vi "HMI.vi"(8 "error in (no error)":errorcluster caption="entrée d'erreur (pas d'erreur)", 11 "Class Popup WaitDIO en entrée":refnum<class "Class Popup WaitVoltage.lvclass">) -> (0 "error out":errorcluster caption="sortie d'erreur", 1 "Input":string, 2 "Operator_Selection":bool, 3 "Class Popup WaitDIO en sortie":refnum<class "Class Popup WaitVoltage.lvclass">)   [LabVIEW 2020, in "Library Instrument & Equipement.lvlib" / "Library Popup.lvlib" / "Class Popup WaitVoltage.lvclass"]
uses:
  Class Popup WaitVoltage.lvclass
  C:/Users/ngarcin/OneDrive - Altyor/Standard TB/Class/Popup/Class Popup (Main)/Class Popup (Main).lvclass
  C:/Users/ngarcin/OneDrive - Altyor/Standard TB/Class/Popup/Class Popup Operator_Validation/Class Popup Operator_Validation (Default)/Class Popup Operator_Validation (Virtual).lvclass
  Commun VI/TypeDef/Liste Error.ctl
  JSON API/JSON Value/Set from JSON string.vi
  Instrument/Instrument (Default)/Class Instrument (Default).lvclass
  JSON API/JSON Value/JSON Value.lvclass
  Class Popup Operator_Validation/Class Popup Operator_Validation (Default)/Class Popup Operator_Validation (Virtual).lvclass
  Class Popup WaitVoltage.lvclass/Class Popup WaitVoltage.ctl
  JSON API/Variant JSON/Variant JSON.lvlib
  JSON API/Get Polymorphic/JSON GetSet.lvlib
  Commun VI/Library Commun.lvlib
panel:
  out "Voltage":dbl format="%#.3g"
  out "Json_String":string
  in  "Bouton NOK":bool caption="Default"
  in  "Bouton OK":bool caption="Validated"
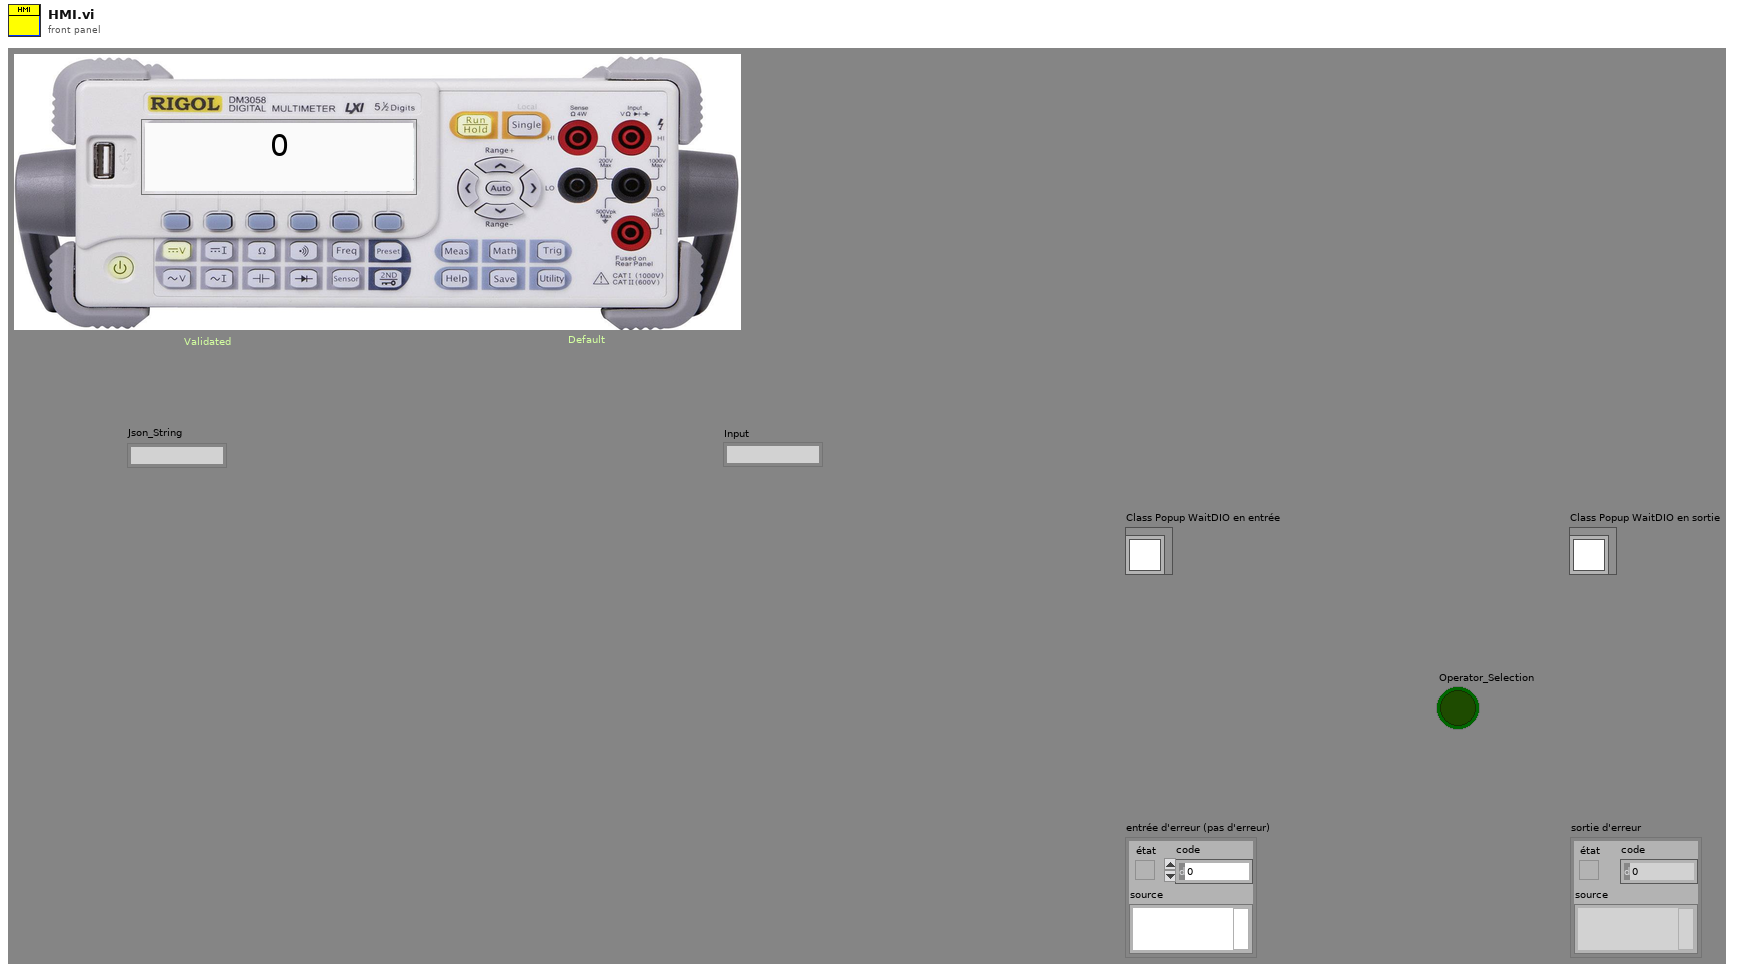
[diagram p1: front panel]
types:
  T1 = cluster{"Instrument":refnum<class "Class Instrument (Default).lvclass">, "Timeout (ms)":u64, "Value Max":dbl, "Value Min":dbl}
  T2 = typedef "Library Commun.lvlib/Liste Error.ctl" = enum16{"Firebase Driver - Get Document", "Firebase Driver - Get Document With Where", "Firebase Driver - Delete Document", "Firebase Driver - Set Document", "Firebase Driver - Update Document", "Firebase Altyor - Search Document Bench", "Firebase Altyor - Class Not in Firebase", "Spectrum_Analyser - Timeout", "Relay Board - Qty Relay", "DIO - Pb Funtion", "Power_Supply - Peripherical not find", "Mutimeter - Peripherical not find", "Instrument - Function Not Used", "Instrument - Instrument name not specified", "Instrument - Allready Initialised", "Instrument - TimeOut", "Instrument - the instrument must be Initialise before", "Instrument - Frame Not received", "Instrument - Frame Nok", "Test - Initialise the File_for_Save", "Test - Timeout", "Test - Cmd Error", "FGV - Variable ", "BDD FireBase - Define Class", "SN - Class Not Define"}
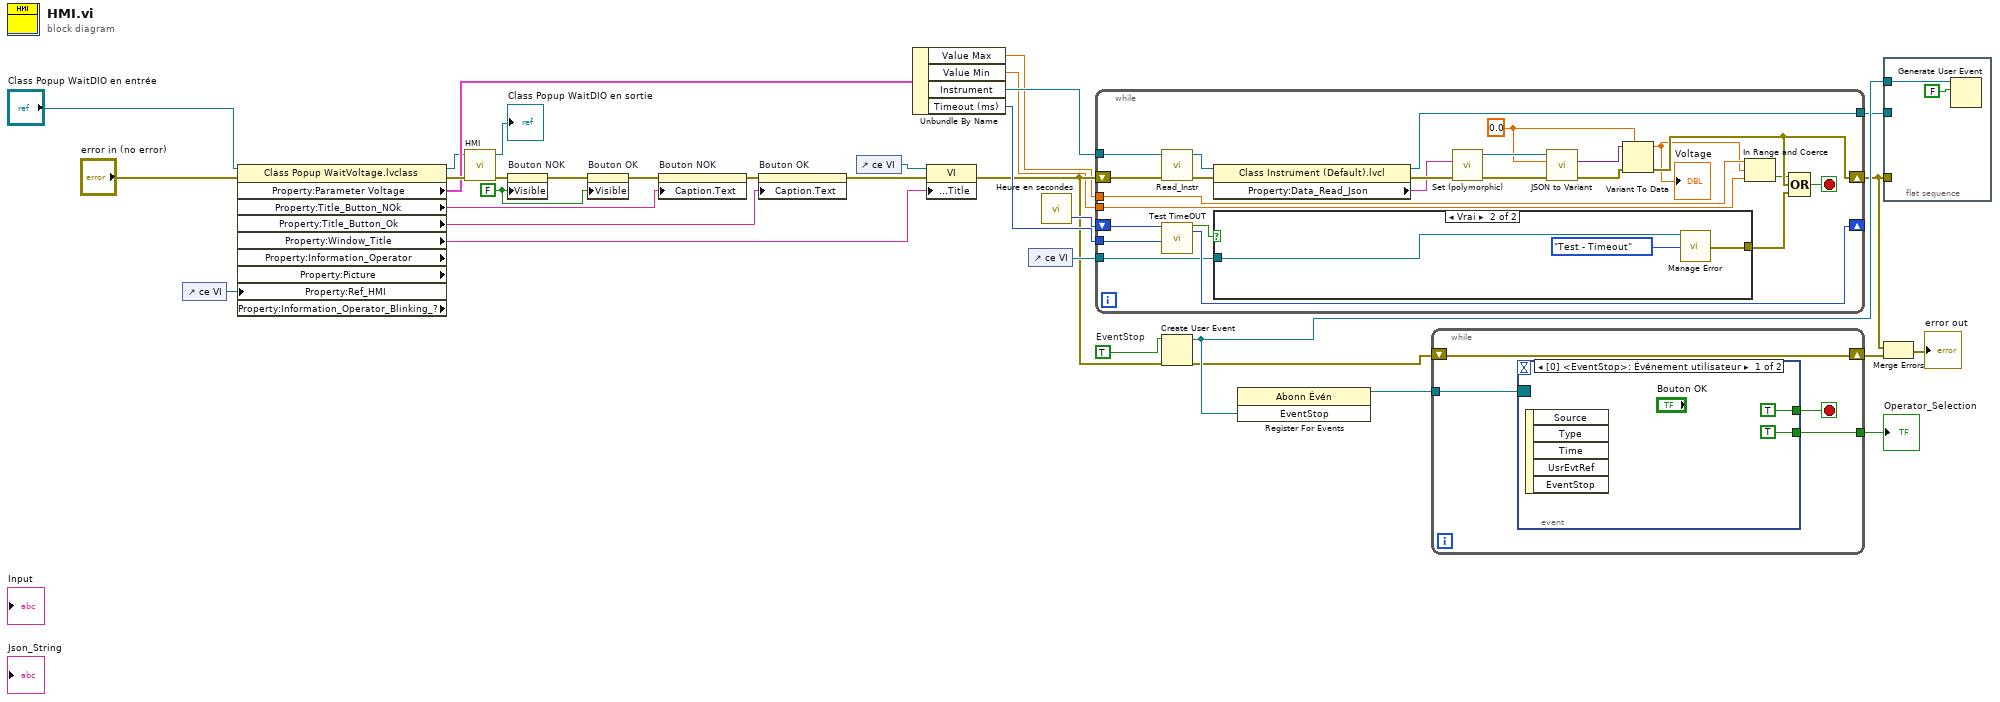
[diagram p0: block diagram]
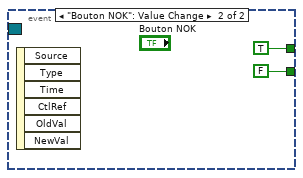
[diagram p3: hidden frame]
diagram:
  w19 = TRUE  # EventStop
  w23 = FALSE ("Visible")
  n1 = control-ref of="ce VI"() -> (w26:refnum<vi>)
  n2 = property class="Class Popup WaitVoltage.lvclass" props=["Property:Parameter Voltage", "Property:Title_Button_NOk", "Property:Title_Button_Ok", "Property:Window_Title", "Property:Information_Operator", "Property:Picture", "Property:Ref_HMI", "Property:Information_Operator_Blinking_?"](reference="Class Popup WaitDIO en entrée", error in="error in (no error)", "Property:Ref_HMI"=w26) -> (reference out=w5:refnum<class "Class Popup WaitVoltage.lvclass">, error out=w13:errorcluster, "Property:Parameter Voltage"=w7:T1, "Property:Title_Button_NOk"=w32:string, "Property:Title_Button_Ok"=w33:string, "Property:Window_Title"=w27:string)  [unwired: 3 out]
  n3 = call-parent "HMI.vi"("error in (no error)"=w13, "Class Popup Operator_Validation (Default) en entrée"=w5) -> ("error out"=w6:errorcluster, "Class Popup Operator_Validation (Default) en sortie"=→"Class Popup WaitDIO en sortie":refnum<class "Class Popup WaitVoltage.lvclass">)  [unwired: 6 in, 2 out]
  n4 = property on="Bouton NOK" class="Bool"(error in=w6, "Visible"=w23) -> (error out=w31:errorcluster)  [unwired: 1 in, 1 out]
  n5 = property on="Bouton OK" class="Bool"(error in=w31, "Visible"=w23) -> (error out=w30:errorcluster)  [unwired: 1 in, 1 out]
  n6 = property on="Bouton NOK" class="Bool"(error in=w30, "Caption.Text"=w32) -> (error out=w29:errorcluster)  [unwired: 1 in, 1 out]
  n7 = property on="Bouton OK" class="Bool"(error in=w29, "Caption.Text"=w33) -> (error out=w12:errorcluster)  [unwired: 1 in, 1 out]
  n8 = control-ref of="ce VI"() -> (w28:refnum<vi>)
  n9 = Unbundle By Name(w7) -> ("Value Max"=w1:dbl, "Value Min"=w2:dbl, "Instrument"=w9:refnum<class "Class Instrument (Default).lvclass">, "Timeout (ms)"=w14:u64)
  n10 = property class="VI"(reference=w28, error in=w12, "Front Panel.Title"=w27) -> (error out=w3:errorcluster)  [unwired: 1 out]
  n11 = control-ref of="ce VI"() -> (w21:refnum<vi>)
  n12 = call "Heure en secondes.vi"() -> ("Heure en milisecondes"=w22:u32)  [unwired: 2 in, 1 out]
  n13 = while {
    tunnel: w9 -> [w57]
    shift-right: [w47] -> w15
    shift-left: w3 -> [w56]
    tunnel: w14 -> [w43]
    shift-right: [w44] -> _
    shift-left: w22 -> [w45]
    tunnel: w21 -> [w42]
    tunnel: [w39] -> w10
    tunnel: w2 -> [w37]
    tunnel: w1 -> [w36]
    stop <- w46 stop-if-true
    w38 = 0.0
    n14 = call-dynamic "Read_Instr.vi"("error in (no error)"=w56, "Class Instrument (Default) en entrée"=w57) -> ("error out"=w48:errorcluster, "Class Instrument (Default) en sortie"=w55:refnum<class "Class Instrument (Default).lvclass">)  [unwired: 8 in]
    n15 = call "Test TimeOUT.vi"("OLD Time"=w45, "TimeOut ms"=w43) -> ("Timeout ?"=w41:bool, "NEW Time"=w44:u32)  [unwired: 13 in, 3 out]
    n16 = property class="Class Instrument (Default).lvcl"(reference=w55, error in=w48) -> (reference out=w39:refnum<class "Class Instrument (Default).lvclass">, error out=w50:errorcluster, "Property:Data_Read_Json"=w49:string)
    n17 = case shown="Vrai" w41 {
      tunnel: w42 -> [_ w59]
      tunnel: [_ w58] -> w40
      frame False {
      }
      frame True {
        n18 = call "Manage Error.vi"("VI in Error"=w59, "Code Erreur"=Liste_Error."Test - Timeout") -> ("error out"=w58:errorcluster)  [unwired: 13 in]
      }
    }
    n19 = call-poly "Set (polymorphic).vi"("error in (no error)"=w50, "JSON stream"=w49) -> ("error out"=w53:errorcluster, "JSON Value out"=w51:refnum<class "JSON Value.lvclass">)  [unwired: 7 in, 1 out]
    n20 = call "JSON to Variant.vi"("error in (no error)"=w53, "Variant (Data Type)"=w38, "JSON Value"=w51) -> ("error out"=w52:errorcluster, "Variant out"=w54:variant)  [unwired: 7 in]
    n21 = Variant To Data(error in=w52, type=w38, Variant=w54) -> (data=w34:dbl, error out=w47:errorcluster)
    "Voltage" <- w34
    n22 = In Range and Coerce(upper limit=w36, x=w34, lower limit=w37) -> (In Range?=w35:bool)  [unwired: 1 out]
    n23 = Compound Arithmetic op=OR ("Opérateur arithmétique")(w35, w47, w40) -> (w46:bool)
  }
  n24 = Create User Event(user event datatype=w19, error in=w3) -> (user event=w18:refnum<user-event>, error out=w11:errorcluster)
  n25 = register-events(w18) -> (reference out=w20:refnum<event-registration>)  [unwired: 2 in, 1 out]
  n26 = while {
    tunnel: [w62] -> w24
    shift-right: [w63] -> w16
    shift-left: w11 -> [w63]
    tunnel: w20 -> [w61]
    stop <- w64 stop-if-true
    n27 = event shown="[0] <EventStop>: Événement utilisateur" {
      selector: w61 -> [_ _]
      dyn-events: _ -> [_ _]
      timeout: _ -> [_ _]
      tunnel: [TRUE ("Valeur (Signalisation)") TRUE ("Valeur (Signalisation)")] -> w64
      tunnel: [TRUE ("Operator_Selection") FALSE ("Operator_Selection")] -> w62
      event User Event {
        n28 = event-data() -> ()  [unwired: 1 in, 5 out]
      }
      event "Bouton NOK": Value Change {
        n29 = event-data() -> ()  [unwired: 1 in, 6 out]
      }
    }
  }
  "Operator_Selection" <- w24
  n30 = flat-sequence {
    tunnel: w18 -> [w70]
    tunnel: w15 -> [_]
    tunnel: w10 -> [_]
    frame #0 {
      n31 = Generate User Event(user event=w70, event data cluster=FALSE ("données d'événement")) -> ()  [unwired: 2 in, 2 out]
    }
  }
  n32 = Merge Errors(w15, w16) -> (→"error out":errorcluster)
